vi "FGV.vi"(2 "S":bool, 3 "A":dbl) -> (0 "T":bool, 1 "B":dbl)   [LabVIEW 2014]
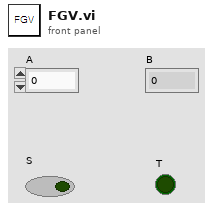
[diagram p1: front panel]
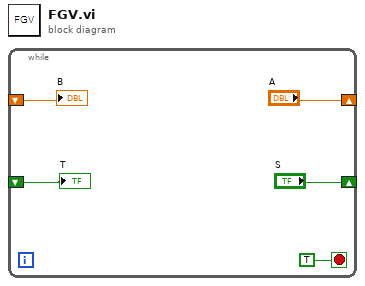
[diagram p0: block diagram]
diagram:
  n1 = while {
    shift-right: ["A"] -> _
    shift-left: _ -> [w2]
    shift-right: ["S"] -> _
    shift-left: _ -> [w1]
    stop <- TRUE stop-if-true
    "B" <- w2
    "T" <- w1
  }
